vi "Parse Main Body.vi"(8 "Error In":errorcluster, 11 "Main Body":string[](array[string])) -> (0 "Error Out":errorcluster, 1 "Provisional Visits":T1 {"TotalSpend" format="£%.2g"; "SpendTaxedA" format="£%.2g"; "SpendTaxedB" format="£%.2g"}, 2 "Main Body Text":string, 3 "Provisional Line Items":T2[](array[typedef]) {"PriceIncDiscount (£)" format="%.2g"; "Discount(£)" format="%.2g"})   [LabVIEW 2018, in "Receipt Parsing.lvlib"]
uses:
  receipt parsing/Receipt Parsing.lvlib
  ReceiptItemInfo.ctl
  database/Visits--cluster.ctl
  database/Items--cluster.ctl
  database/Database.lvlib
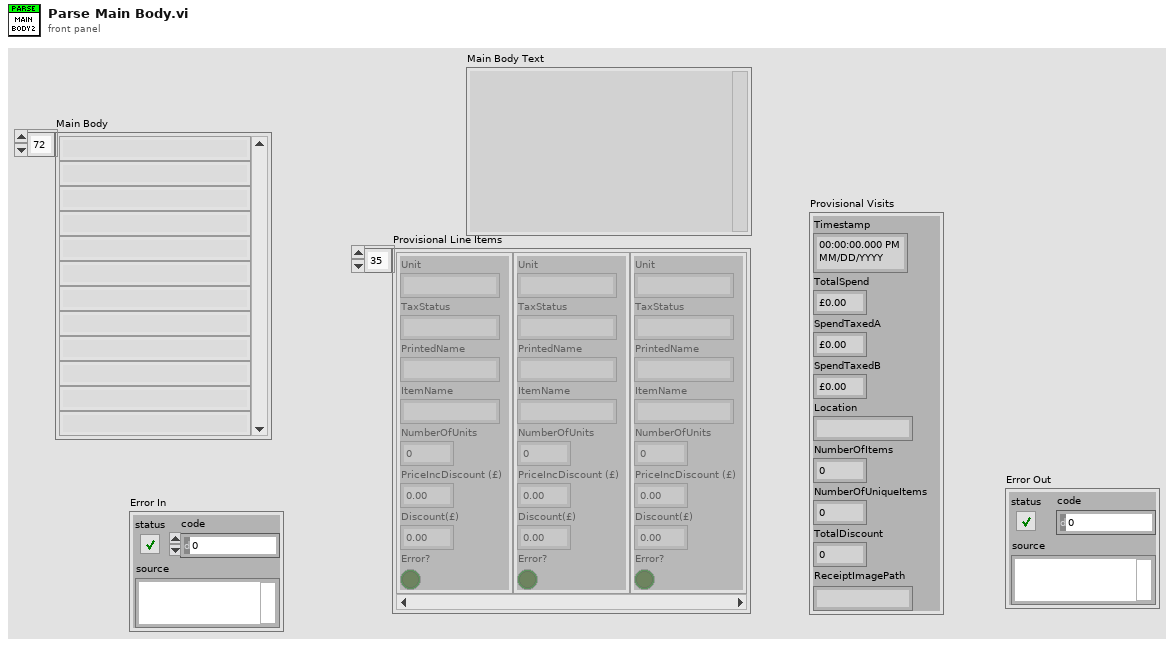
[diagram p1: front panel]
types:
  T1 = typedef "Database.lvlib/Visits--cluster.ctl" = cluster{"Timestamp":timestamp, "TotalSpend":dbl, "SpendTaxedA":dbl, "SpendTaxedB":dbl, "Location":string, "NumberOfItems":i32, "NumberOfUniqueItems":i32, "TotalDiscount":dbl, "ReceiptImagePath":string}
  T2 = typedef "Receipt Parsing.lvlib/ReceiptItemInfo.ctl" = cluster{"Unit":string, "TaxStatus":string, "PrintedName":string, "ItemName":string, "NumberOfUnits":i32, "PriceIncDiscount (£)":dbl, "Discount(£)":dbl, "Error?":bool}
  T3 = typedef "Database.lvlib/Items--cluster.ctl" = cluster{"ItemName":string, "PrintedNames":string, "TaxStatus":string, "Unit":string, "IsFood":bool, "IsVeg":bool, "IsFavourite":bool}
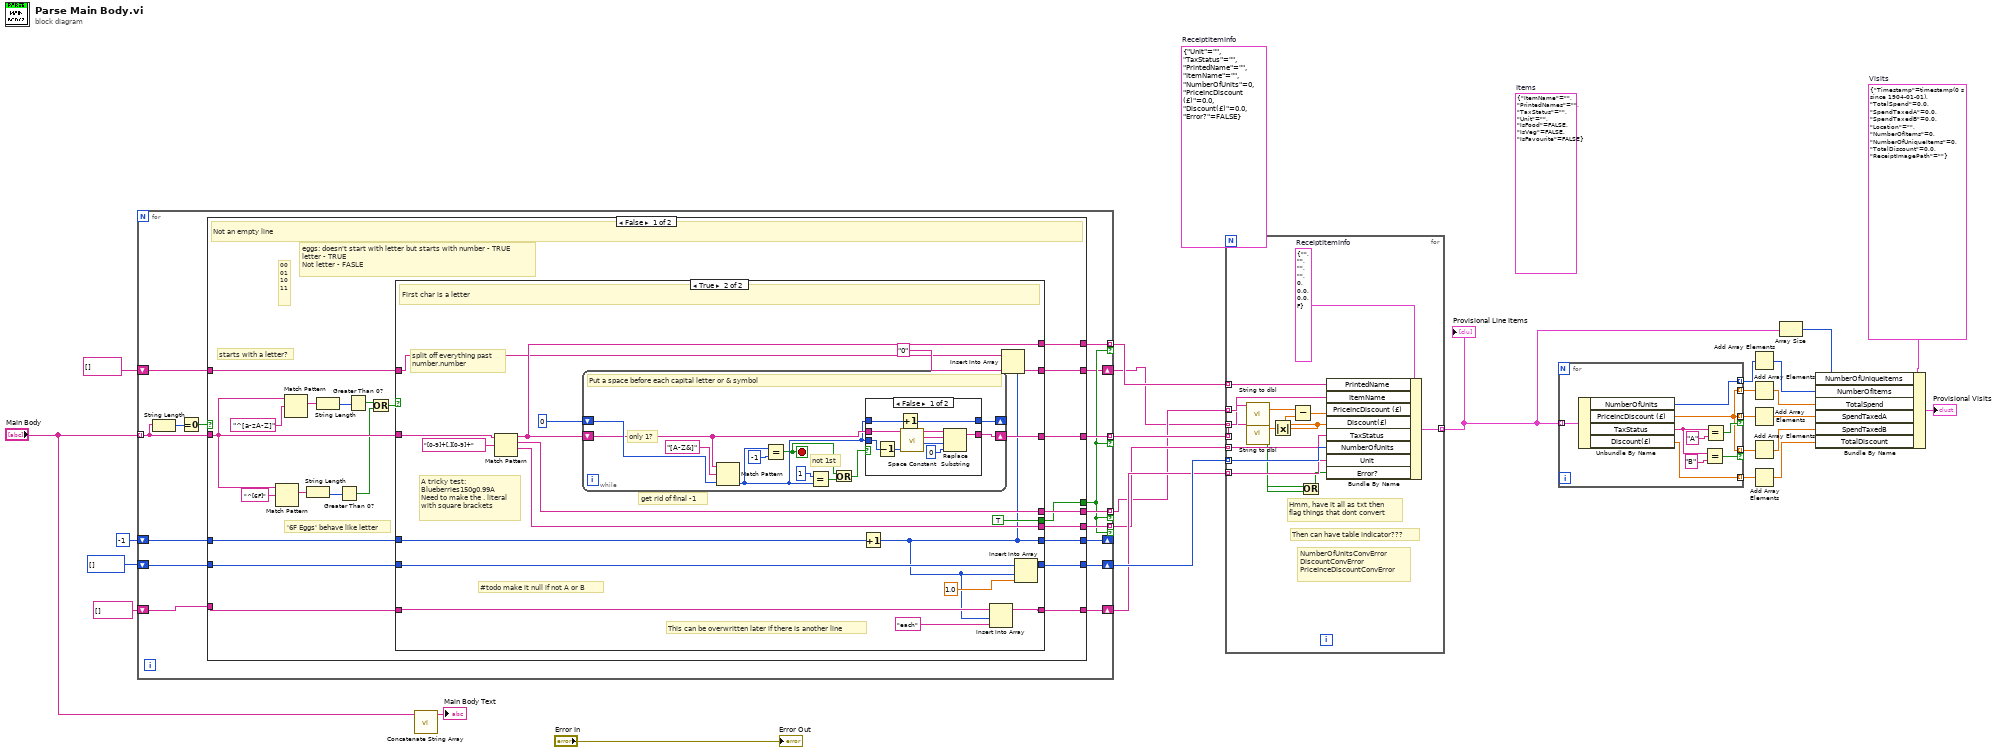
[diagram p0: block diagram]
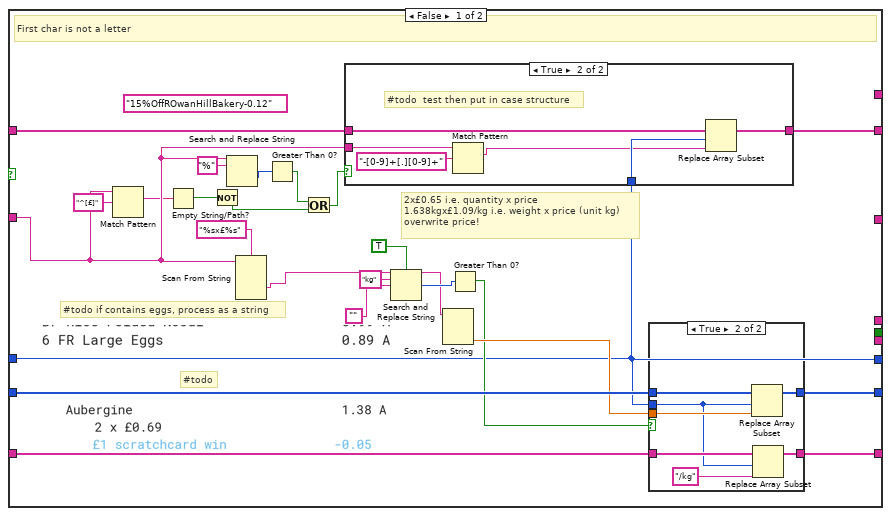
[diagram p2: hidden frame]
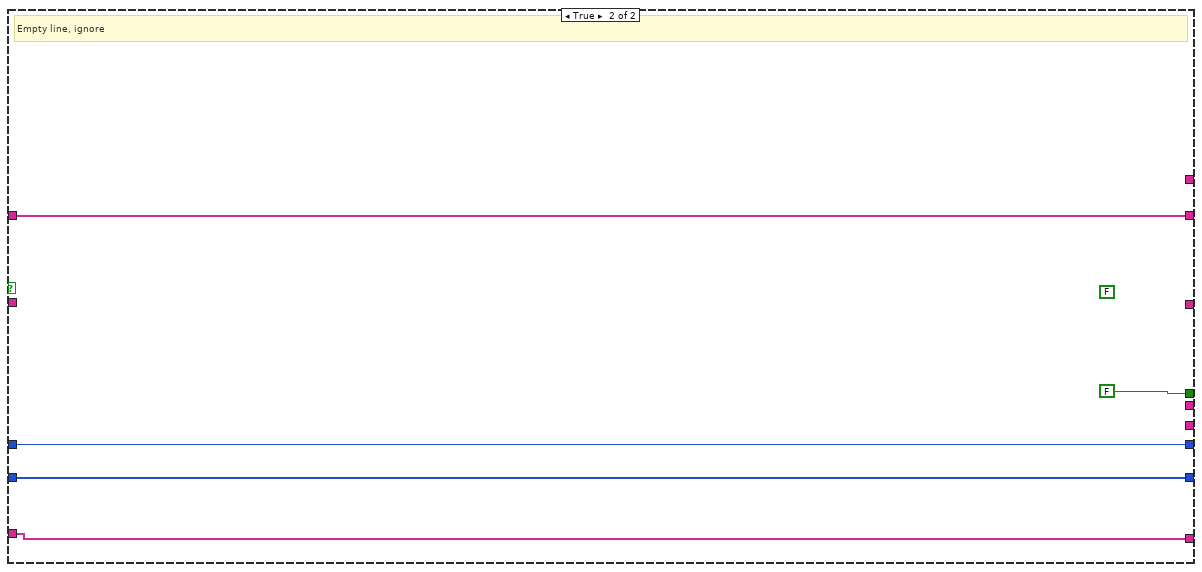
[diagram p6: hidden frame]
diagram:
  (unwired) T3 {"ItemName"="", "PrintedNames"="", "TaxStatus"="", "Unit"="", "IsFood"=FALSE, "IsVeg"=FALSE, "IsFavourite"=FALSE}  # Items
  w8 = T1 {"Timestamp"=timestamp(0 s since 1904-01-01), "TotalSpend"=0.0, "SpendTaxedA"=0.0, "SpendTaxedB"=0.0, "Location"="", "NumberOfItems"=0, "NumberOfUniqueItems"=0, "TotalDiscount"=0.0, "ReceiptImagePath"=""}  # Visits
  (unwired) T2 {"Unit"="", "TaxStatus"="", "PrintedName"="", "ItemName"="", "NumberOfUnits"=0, "PriceIncDiscount (£)"=0.0, "Discount(£)"=0.0, "Error?"=FALSE}  # ReceiptItemInfo
  n1 = for {
    tunnel: "Main Body" -> [w42] mode=indexing
    tunnel: [w44] -> w20 mode=indexing if=w31
    tunnel: [w43] -> w16 mode=indexing if=w31
    tunnel: [w39] -> w21 mode=indexing if=w31
    tunnel: [w38] -> w17 mode=indexing if=w31
    shift-right: [w37] -> w19
    shift-left: i32[] [] -> [w36]
    shift-right: [w34] -> _
    shift-left: -1 -> [w35]
    shift-right: [w33] -> w18
    shift-left: string[] [] -> [w32]
    shift-right: [w30] -> w15
    shift-left: string[] [] -> [w29]
    n2 = String Length(string=w42) -> (length=w41:i32)
    n3 = Equal To 0?(x=w41) -> (x = 0?=w40:bool)
    n4 = case shown="False" w40 {
      tunnel: [w67 _] -> w44
      tunnel: [w66 _] -> w43
      tunnel: w42 -> [w50 _]
      tunnel: [w62 FALSE] -> w31
      tunnel: [w61 _] -> w39
      tunnel: [w60 _] -> w38
      tunnel: [w57 w152] -> w37
      tunnel: w36 -> [w56 w152]
      tunnel: w35 -> [w58 w151]
      tunnel: [w59 w151] -> w34
      tunnel: [w55 w150] -> w33
      tunnel: w32 -> [w54 w150]
      tunnel: [w53 w149] -> w30
      tunnel: w29 -> [w52 w149]
      frame False {
        # "eggs: doesn't start with letter but starts with number - TRUE\nletter - TRUE\nNot letter - FASLE"
        # "00\n01\n10\n11"
        # "'6F Eggs' behave like letter"
        # "starts with a letter?"
        # "Not an empty line"
        n5 = Match Pattern(string=w50, regular expression="^[6F]") -> (match substring=w49:string)  [unwired: 1 in, 3 out]
        n6 = Match Pattern(string=w50, regular expression="^[a-zA-Z]") -> (match substring=w63:string)  [unwired: 1 in, 3 out]
        n7 = String Length(string=w49) -> (length=w46:i32)
        n8 = String Length(string=w63) -> (length=w65:i32)
        n9 = Greater Than 0?(x=w46) -> (x > 0?=w45:bool)
        n10 = Greater Than 0?(x=w65) -> (x > 0?=w48:bool)
        n11 = Or(x=w48, y=w45) -> (x .or. y?=w47:bool)
        n12 = case shown="True" w47 {
          tunnel: w50 -> [w74 w125]
          tunnel: [_ w126] -> w67
          tunnel: [_ w123] -> w66
          tunnel: [_ TRUE] -> w62
          tunnel: [_ w121] -> w61
          tunnel: [_ w120] -> w60
          tunnel: [w75 w109] -> w59
          tunnel: w58 -> [w75 w119]
          tunnel: [w84 w118] -> w57
          tunnel: w56 -> [w85 w117]
          tunnel: [w82 w115] -> w55
          tunnel: w54 -> [w81 w114]
          tunnel: [w77 w112] -> w53
          tunnel: w52 -> [w76 w110]
          frame False {
            (unwired) "15%OffROwanHillBakery-0.12"
            # "#todo"
            # "#todo if contains eggs, process as a string"
            # "2x£0.65 i.e. quantity x price\n1.638kgx£1.09/kg i.e. weight x price (unit kg)\noverwrite price!"
            # "First char is not a letter"
            n13 = Match Pattern(string=w74, regular expression="^[£]") -> (match substring=w72:string)  [unwired: 1 in, 3 out]
            n14 = Empty String/Path?(string/path=w72) -> (empty?=w71:bool)
            n15 = Not(x=w71) -> (.not. x?=w69:bool)
            n16 = Search and Replace String(input string=w74, search string="%") -> (offset past replacement=w78:i32)  [unwired: 6 in, 3 out]
            n17 = Scan From String(format string="%sx£%s", input string=w74) -> (output 1=w90:string)  [unwired: 5 in, 3 out]
            n18 = Greater Than 0?(x=w78) -> (x > 0?=w70:bool)
            n19 = Or(x=w70, y=w69) -> (x .or. y?=w68:bool)
            n20 = case shown="True" w68 {
              tunnel: w74 -> [_ w98]
              tunnel: [w93 w97] -> w77
              tunnel: w76 -> [w93 w96]
              tunnel: w75 -> [_ w95]
              frame False {
              }
              frame True {
                # "#todo  test then put in case structure"
                n21 = Match Pattern(string=w98, regular expression="-[0-9]+[.][0-9]+") -> (match substring=w94:string)  [unwired: 1 in, 3 out]
                n22 = Replace Array Subset(array=w96, new element=w94, index=w95) -> (w97:string[])
              }
            }
            n23 = Search and Replace String(case sensitive?=TRUE ("ignore case? (F)"), input string=w90, search string="kg", replace string="") -> (result string=w86:string, number of replacements=w88:i32)  [unwired: 4 in, 2 out]
            n24 = Scan From String(input string=w86) -> (output 1=w83:dbl)  [unwired: 4 in, 3 out]
            n25 = Greater Than 0?(x=w88) -> (x > 0?=w80:bool)
            n26 = case shown="True" w80 {
              tunnel: w85 -> [w100 w108]
              tunnel: [w100 w107] -> w84
              tunnel: w83 -> [_ w106]
              tunnel: w75 -> [_ w102]
              tunnel: [w101 w104] -> w82
              tunnel: w81 -> [w101 w103]
              frame False {
              }
              frame True {
                n27 = Replace Array Subset(array=w108, new element=w106, index=w102) -> (w107:i32[])
                n28 = Replace Array Subset(array=w103, new element="/kg" ("search string"), index=w102) -> (w104:string[])
              }
            }
          }
          frame True {
            # "A tricky test:\nBlueberries150g0.99A\nNeed to make the . literal\nwith square brackets"
            # "This can be overwritten later if there is another line"
            # "#todo make it null if not A or B"
            # "split off everything past\nnumber.number"
            # "get rid of final -1"
            # "First char is a letter"
            n29 = Match Pattern(string=w125, regular expression="[0-9]+[.][0-9]+") -> (before substring=w121:string, match substring=w123:string, after substring=w120:string)  [unwired: 1 in, 1 out]
            n30 = while {
              shift-right: [w133] -> _
              shift-left: 0 ("offset past match") -> [w136]
              shift-right: [w135] -> w126
              shift-left: w121 -> [w134]
              stop <- w129 stop-if-true
              # "not 1st"
              # "only 1?"
              # "Put a space before each capital letter or & symbol"
              n31 = Match Pattern(string=w134, regular expression="[A-Z&]", offset (0)=w136) -> (offset past match=w131:i32)  [unwired: 3 out]
              n32 = Equal?(x=w131, y=-1) -> (x = y?=w129:bool)
              n33 = Equal?(x=1, y=w131) -> (x = y?=w132:bool)
              n34 = Or(x=w129, y=w132) -> (x .or. y?=w130:bool)
              n35 = case shown="False" w130 {
                tunnel: w131 -> [w143 _]
                tunnel: [w145 w148] -> w135
                tunnel: w134 -> [w144 w148]
                tunnel: w131 -> [w140 w147]
                tunnel: [w139 w147] -> w133
                frame False {
                  n36 = Decrement(x=w143) -> (x-1=w142:i32)
                  n37 = Increment(x=w140) -> (x+1=w139:i32)
                  n38 = call <vilib>:"Space Constant.vi"() -> ("String"=w146:string)
                  n39 = Replace Substring(2:0 ("length (len. of substring)"), 3:w142, 4:w146, 5:w144) -> (1:w145:string)  [unwired: 1 out]
                }
                frame True {
                }
              }
            }
            n40 = Increment(x=w119) -> (x+1=w109:i32)
            n41 = Insert Into Array(array=w114, index=w109, new element="each" ("new element/subarray")) -> (w115:string[])
            n42 = Insert Into Array(array=w110, index=w109, new element="0" ("Read String")) -> (w112:string[])
            n43 = Insert Into Array(array=w117, index=w109, new element=1.0) -> (w118:i32[])
          }
        }
      }
      frame True {
        (unwired) FALSE
        # "Empty line, ignore"
      }
    }
  }
  n44 = call "Concatenate String Array.vi"("Array"="Main Body") -> ("Concatenated String"=→"Main Body Text":string)  [unwired: 10 in]
  n45 = for {
    tunnel: w21 -> [w168] mode=indexing
    tunnel: w20 -> [w162] mode=indexing
    tunnel: w19 -> [w167] mode=indexing
    tunnel: w18 -> [w166] mode=indexing
    tunnel: w17 -> [w165] mode=indexing
    tunnel: [w164] -> w14 mode=indexing
    tunnel: w16 -> [w163] mode=indexing
    tunnel: w15 -> [w161] mode=indexing
    w169 = T2 {"Unit"="", "TaxStatus"="", "PrintedName"="", "ItemName"="", "NumberOfUnits"=0, "PriceIncDiscount (£)"=0.0, "Discount(£)"=0.0, "Error?"=FALSE}  # ReceiptItemInfo
    # "Then can have table indicator???"
    # "NumberOfUnitsConvError\nDiscountConvError\nPriceInceDiscountConvError"
    # "Hmm, have it all as txt then\nflag things that dont convert"
    n46 = call "String to dbl.vi"("String"=w163) -> ("Error?"=w158:bool, "dbl"=w160:dbl)  [unwired: 9 in]
    n47 = call "String to dbl.vi"("String"=w161) -> ("Error?"=w157:bool, "dbl"=w155:dbl)  [unwired: 9 in]
    n48 = Absolute Value(x=w155) -> (abs(x)=w154:dbl)
    n49 = Subtract(x=w160, y=w154) -> (x-y=w159:dbl)
    n50 = Or(x=w158, y=w157) -> (x .or. y?=w156:bool)
    n51 = Bundle By Name(cluster=w169, "PrintedName"=w168, "ItemName"=w162, "PriceIncDiscount (£)"=w159, "Discount(£)"=w154, "TaxStatus"=w165, "NumberOfUnits"=w167, "Unit"=w166, "Error?"=w156) -> (w164:T2)
  }
  "Provisional Line Items" <- w14
  n52 = for {
    tunnel: w14 -> [w178] mode=indexing
    tunnel: [w177] -> w11 mode=indexing
    tunnel: [w170] -> w13 mode=indexing if=w172
    tunnel: [w170] -> w12 mode=indexing if=w173
    tunnel: [w171] -> w10 mode=indexing
    tunnel: [w170] -> w9 mode=indexing
    n53 = Unbundle By Name(w178) -> ("NumberOfUnits"=w177:i32, "PriceIncDiscount (£)"=w170:dbl, "TaxStatus"=w175:string, "Discount(£)"=w171:dbl)
    n54 = Equal?(x=w175, y="B") -> (x = y?=w173:bool)
    n55 = Equal?(x=w175, y="A") -> (x = y?=w172:bool)
  }
  n56 = Add Array Elements(numeric array=w11) -> (sum=w6:i32)
  n57 = Add Array Elements(numeric array=w9) -> (sum=w5:dbl)
  n58 = Add Array Elements(numeric array=w13) -> (sum=w4:dbl)
  n59 = Add Array Elements(numeric array=w12) -> (sum=w3:dbl)
  n60 = Add Array Elements(numeric array=w10) -> (sum=w2:dbl)
  n61 = Array Size(array=w14) -> (size(s)=w7:i32)
  n62 = Bundle By Name(cluster=w8, "NumberOfUniqueItems"=w7, "NumberOfItems"=w6, "TotalSpend"=w5, "SpendTaxedA"=w4, "SpendTaxedB"=w3, "TotalDiscount"=w2) -> (→"Provisional Visits":T1)
  "Error Out" <- "Error In"
